vi "Messy.vi"() -> ()   [LabVIEW 2010]
doc: "A sample VI demonstrating a pooly designed front panel and block diagram."
panel:
  out "Numeric 6":dbl
  in  "Numeric 5":dbl
  in  "Numeric 4":dbl
  out "Numeric 3":dbl
  in  "Numeric 2":dbl
  in  "Numeric 1":dbl
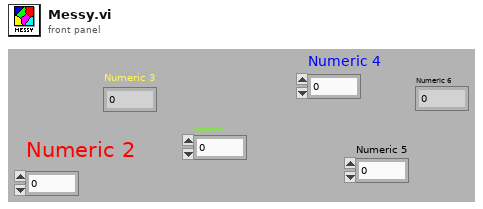
[diagram p1: front panel]
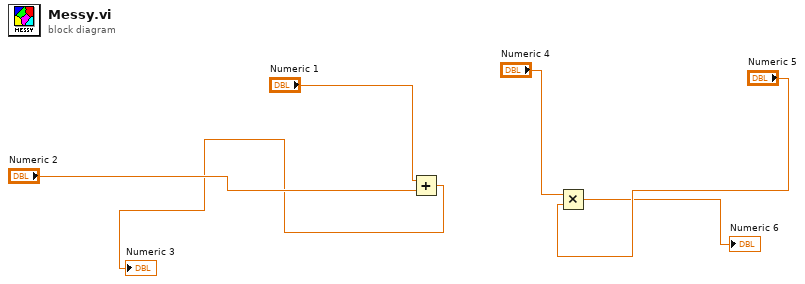
[diagram p0: block diagram]
diagram:
  n1 = Add(x="Numeric 1", y="Numeric 2") -> (x+y=→"Numeric 3":dbl)
  n2 = Multiply(x="Numeric 4", y="Numeric 5") -> (x*y=→"Numeric 6":dbl)
